vi "RGB to HSV.vi"(9 "b in":dbl, 10 "g in":dbl, 11 "r in":dbl) -> (1 "[2]":dbl, 2 "[1]":dbl, 3 "[0]":dbl)   [LabVIEW 2017]
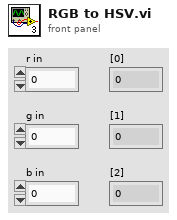
[diagram p1: front panel]
types:
  T1 = cluster{"[0]":dbl, "[1]":dbl, "[2]":dbl, "[3]":dbl, "[4]":dbl, "[5]":dbl, "[6]":dbl, "[7]":dbl, "[8]":dbl}
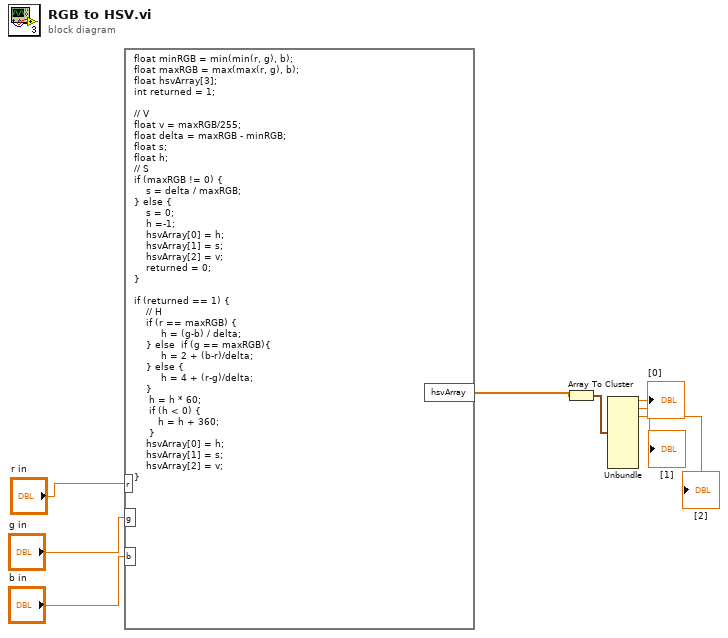
[diagram p0: block diagram]
diagram:
  n1 = formula code="float minRGB = min(min(r, g), b);\nfloat maxRGB = max(max(r, g), b);\nfloat hsvArray[3];\nint returned = 1;\n \n// V\nfloat v = maxRGB/255;\nfloat delta = maxRGB - minRGB;\nfloat s;\nfloat h;\n// S\nif (maxRGB != 0) {\n    s = delta / maxRGB;\n} else {\n    s = 0;\n    h =-1;\n    hsvArray[0] = h;\n    hsvArray[1] = s;\n    hsvArray[2] = v;\n    returned = 0;\n}\n\nif (returned == 1) {\n    // H\n    if (r == maxRGB) {\n         h = (g-b) / delta;\n    } else  if (g == maxRGB){\n         h = 2 + (b-r)/delta;\n    } else {\n         h = 4 + (r-g)/delta;\n    }\n     h = h * 60;\n     if (h < 0) {\n        h = h + 360;\n     }\n    hsvArray[0] = h;\n    hsvArray[1] = s;\n    hsvArray[2] = v;\n}"("r"="r in", "g"="g in", "b"="b in") -> ("hsvArray"=w4:dbl[])
  n2 = Array To Cluster(array=w4) -> (cluster=w5:T1)
  n3 = Unbundle(w5) -> ("[0]"=→"[0]":dbl, "[1]"=→"[1]":dbl, "[2]"=→"[2]":dbl)  [unwired: 6 out]
